vi "Load AI Driver.vi"(8 "error in (no error)":errorcluster, 9 "Config Path":path, 10 "Section":string, 11 "abstract IO Factory in":refnum<class "abstract IO Factory.lvclass">) -> (0 "error out":errorcluster, 2 "AI Driver.lvclass":refnum<class "AI Driver.lvclass">)   [LabVIEW 2022 SP3, in "abstract IO Factory.lvclass"]
uses:
  abstract IO Factory.lvclass
  AI Driver/AI Driver.lvclass
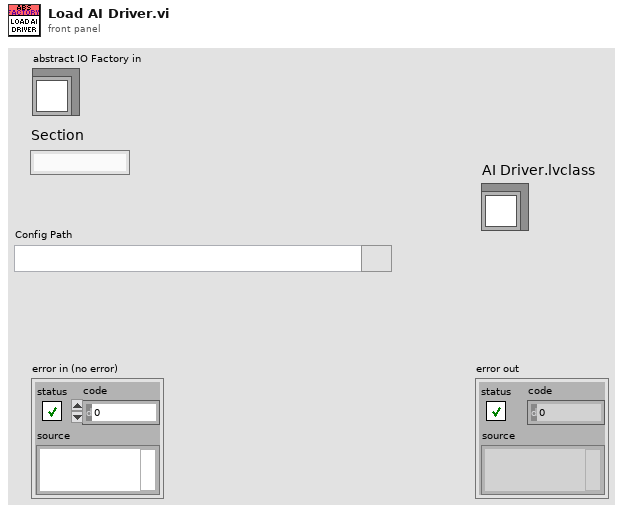
[diagram p1: front panel]
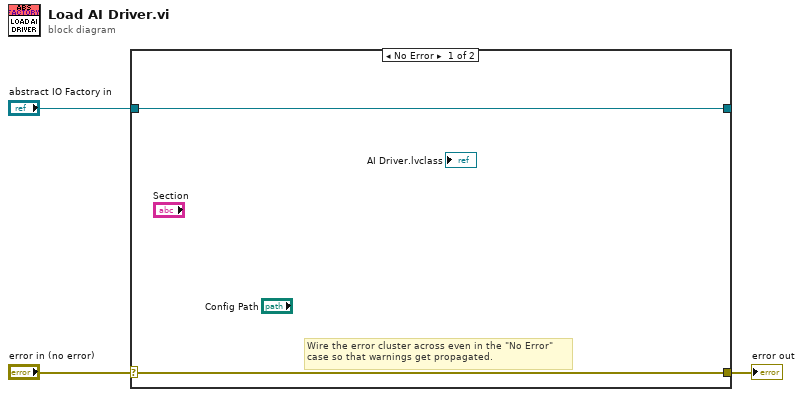
[diagram p0: block diagram]
diagram:
  n1 = case shown="No Error" "error in (no error)" {
    selector: "error in (no error)" -> [w4 w7]
    tunnel: [w4 w7] -> w2
    tunnel: [w5 w6] -> _
    tunnel: "abstract IO Factory in" -> [w5 w6]
    frame No Error {
      # "Wire the error cluster across even in the \"No Error\"\ncase so that warnings get propagated."
    }
    frame Error {
    }
  }
  "error out" <- w2
